vi "NI Switch Disconnect All.vi"(8 "error in (no error)":errorcluster, 11 "RelayOutput in":refnum<class "NISwitch.lvclass">) -> (0 "error out":errorcluster, 3 "RelayOutput out":refnum<class "NISwitch.lvclass">)   [LabVIEW 2023, in "HardwareAbstractionLayer_LVOOP.lvlib" / "NISwitch.lvclass"]
uses:
  NISwitch.lvclass
  NISwitch.lvclass/NISwitch.ctl
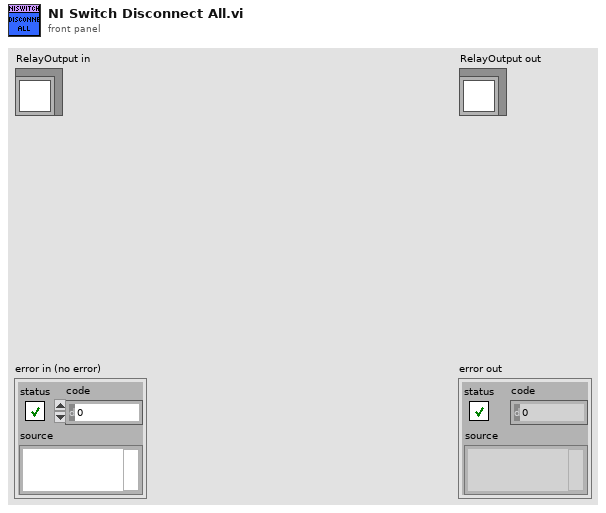
[diagram p1: front panel]
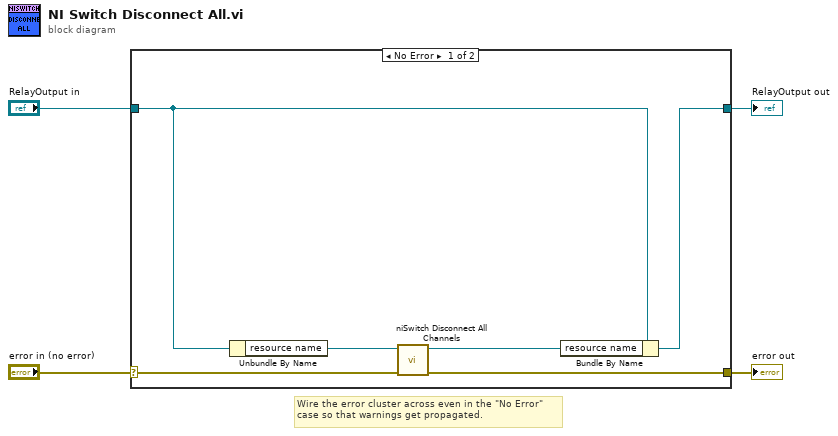
[diagram p0: block diagram]
diagram:
  # "Wire the error cluster across even in the \"No Error\"\ncase so that warnings get propagated."
  n1 = case shown="No Error" "error in (no error)" {
    selector: "error in (no error)" -> [w10 w12]
    tunnel: [w9 w12] -> w3
    tunnel: [w6 w11] -> w1
    tunnel: "RelayOutput in" -> [w7 w11]
    frame No Error {
      n2 = Unbundle By Name(w7) -> ("resource name"=w8:refnum<k15>)
      n3 = call <instrlib>:"niSwitch Disconnect All Channels.vi"("error in (no error)"=w10, "instrument handle"=w8) -> ("error out"=w9:errorcluster, "instrument handle out"=w5:refnum<k15>)  [unwired: 8 in]
      n4 = Bundle By Name(cluster=w7, "resource name"=w5) -> (w6:refnum<class "NISwitch.lvclass">)
    }
    frame Error {
    }
  }
  "error out" <- w3
  "RelayOutput out" <- w1
